vi "new_P11.vi"(4 "Boolean":bool, 6 "P31":fxp<+,32,16>, 7 "P11":fxp<+,32,16>, 8 "E11":fxp<+,32,16>, 9 "feedback_time (ms)":fxp<+,16,1>, 10 "P13":fxp<+,32,16>, 11 "P33":fxp<+,32,16>) -> (2 "output valid":bool, 3 "P11+dt*P31 + dt*(P13+dt*P33) + E1":fxp<+,32,16>)   [LabVIEW 2020]
uses:
  <vilib>/rvi/FXPMathLib/FxpMul/XNode/nifxpmath_Multiplier.xnode
  <vilib>/rvi/FXPMathLib/FxpAdd/XNode/nifxpmath_Add.xnode
  <vilib>/rvi/FXPMathLib/sim/FxpSim.dll
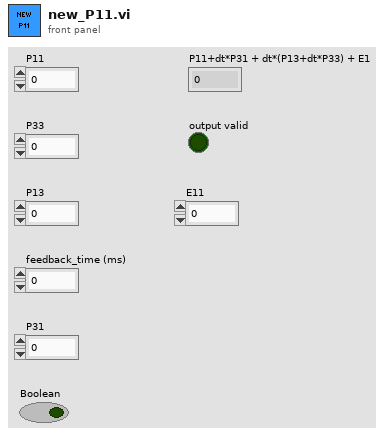
[diagram p1: front panel]
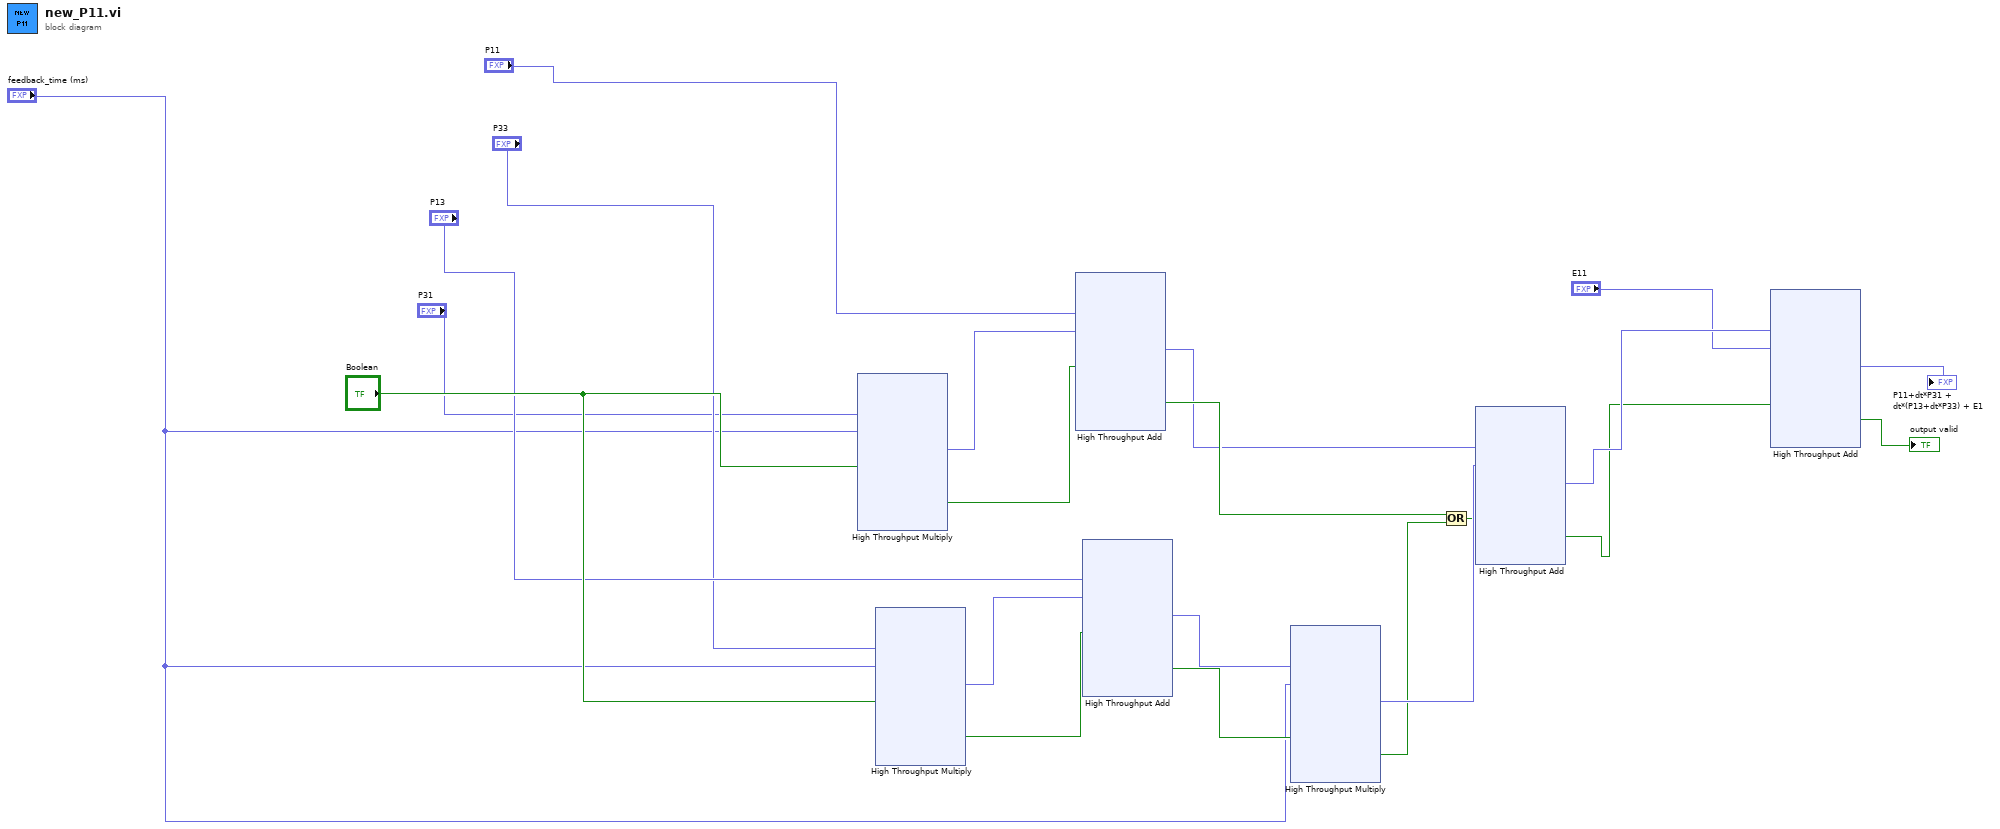
[diagram p0: block diagram]
diagram:
  n1 = xnode "High Throughput Multiply"("x"="P31", "y"="feedback_time (ms)", "input valid"="Boolean") -> ("x*y"=w9:fxp<+,32,16>, "output valid"=w15:bool)  [unwired: 1 in, 1 out]
  n2 = xnode "High Throughput Multiply"("x"="P33", "y"="feedback_time (ms)", "input valid"="Boolean") -> ("x*y"=w11:fxp<+,32,16>, "output valid"=w16:bool)  [unwired: 1 in, 1 out]
  n3 = xnode "High Throughput Add"("x"="P11", "y"=w9, "input valid"=w15) -> ("x+y"=w13:fxp<+,32,16>, "output valid"=w17:bool)  [unwired: 1 in, 1 out]
  n4 = xnode "High Throughput Add"("x"="P13", "y"=w11, "input valid"=w16) -> ("x+y"=w19:fxp<+,32,16>, "output valid"=w20:bool)  [unwired: 1 in, 1 out]
  n5 = xnode "High Throughput Multiply"("x"=w19, "y"="feedback_time (ms)", "input valid"=w20) -> ("x*y"=w22:fxp<+,32,16>, "output valid"=w21:bool)  [unwired: 1 in, 1 out]
  n6 = Or(x=w17, y=w21) -> (x .or. y?=w18:bool)
  n7 = xnode "High Throughput Add"("x"=w13, "y"=w22, "input valid"=w18) -> ("x+y"=w5:fxp<+,32,16>, "output valid"=w2:bool)  [unwired: 1 in, 1 out]
  n8 = xnode "High Throughput Add"("x"=w5, "y"="E11", "input valid"=w2) -> ("x+y"=→"P11+dt*P31 + dt*(P13+dt*P33) + E1":fxp<+,32,16>, "output valid"=→"output valid":bool)  [unwired: 1 in, 1 out]
